vi "Wait for Nested Actors to shutdown.vi"(8 "error in (no error)":errorcluster, 9 "Timeout (-1)":i32=-1, 11 "Syringe Line in":refnum<class "Syringe Line.lvclass">) -> (0 "error out":errorcluster, 3 "Syringe Line out":refnum<class "Syringe Line.lvclass">)   [LabVIEW 2015, in "cRIO-Carbondioxide.lvlib" / "CO2-Actor.lvlib" / "Syringe Line.lvclass"]
uses:
  Syringe Line.lvclass
  CO2 Actor/CO2 Actor.lvclass
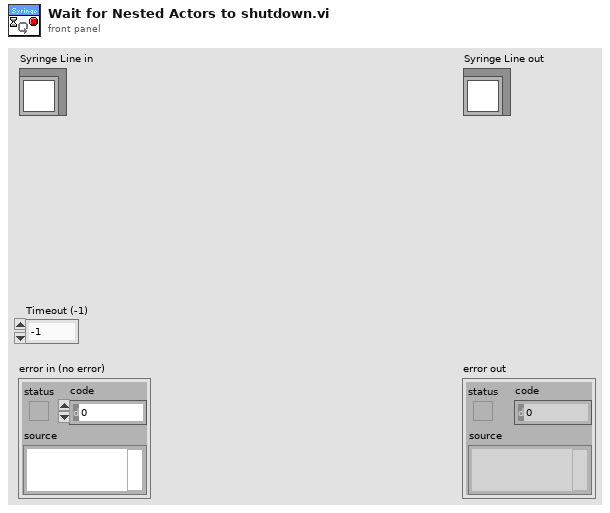
[diagram p1: front panel]
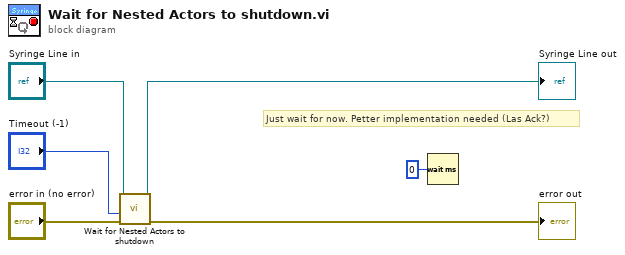
[diagram p0: block diagram]
diagram:
  # "Just wait for now. Petter implementation needed (Las Ack?)"
  n1 = call-parent "Wait for Nested Actors to shutdown.vi"("error in (no error)"="error in (no error)", "Timeout (-1)"="Timeout (-1)", "CO2 Actor in"="Syringe Line in") -> ("error out"=→"error out":errorcluster, "CO2 Actor out"=→"Syringe Line out":refnum<class "Syringe Line.lvclass">)  [unwired: 7 in]
  n2 = Wait (ms)(milliseconds to wait=u32 0) -> ()  [unwired: 1 out]
